vi "Demo.vi"() -> ()   [LabVIEW 2020, in "BlueVariantViewDemo.lvlib"]
uses:
  BlueVariantViewDemo.lvlib
  Classes/Child/Child.lvclass
  C:/DSCE code/Serialization OpenSource/BlueVariantView/Source/Demo/Classes/Parent/Parent.lvclass
  API/Typedefs/Options.ctl
  API/Typedefs/ValueOptions.ctl
  Classes/Parent/Parent.lvclass/Parent.ctl
  Classes/Child/Child.lvclass/Child.ctl
  Classes/Parent/Write connection ID.vi
  Classes/Parent/Write Name.vi
  Classes/Child/Write Color.vi
  Classes/Child/Write Port.vi
  Classes/Child/Write timeout.vi
  BlueVariantView.lvlib
panel:
  out "error out":errorcluster
  in  "Config":T1={"RS232"={"baud rate"=9600, "data bits"=8, "parity"=enum."Even", "stop bits"=10, "flow control"=3, "Numeric"=0.0, "MyRing"=0}, "LEDs"=[FALSE, TRUE, TRUE], "Hazzards"=[{"Alarm"=FALSE, "level"=0.0, "states"=[1, 2, 3]}, {"Alarm"=TRUE, "level"=2.0, "states"=[3, 0, 3, 1]}, {"Alarm"=TRUE, "level"=0.0, "states"=[]}], "Calibration"=[[1.0, 1.2], [2.0, 2.3], [3.0, 3.4]], "MyError"={"status"=FALSE, "code"=123, "source"="This is an error"}, "MyMap"={}, "MySet"={}, "MyVariant"=variant, "MyDVR"=refnum, "MyObject"=refnum, "current time"=timestamp(0 s since 1904-01-01)} {"RS232"."MyRing" items=["a"=3, "b"=4]; "RS232"."flow control" items=["None", "XON/XOFF", "RTS/CTS", "XON/XOFF & RTS/CTS", "DTR/DSR", "XON/XOFF & DTR/DSR"]; "RS232"."stop bits" items=["1.0"=10, "1.5"=15, "2.0"=20]; "RS232"."data bits" min=5 max=8 step=1}
  in  "Tree":string(tree)
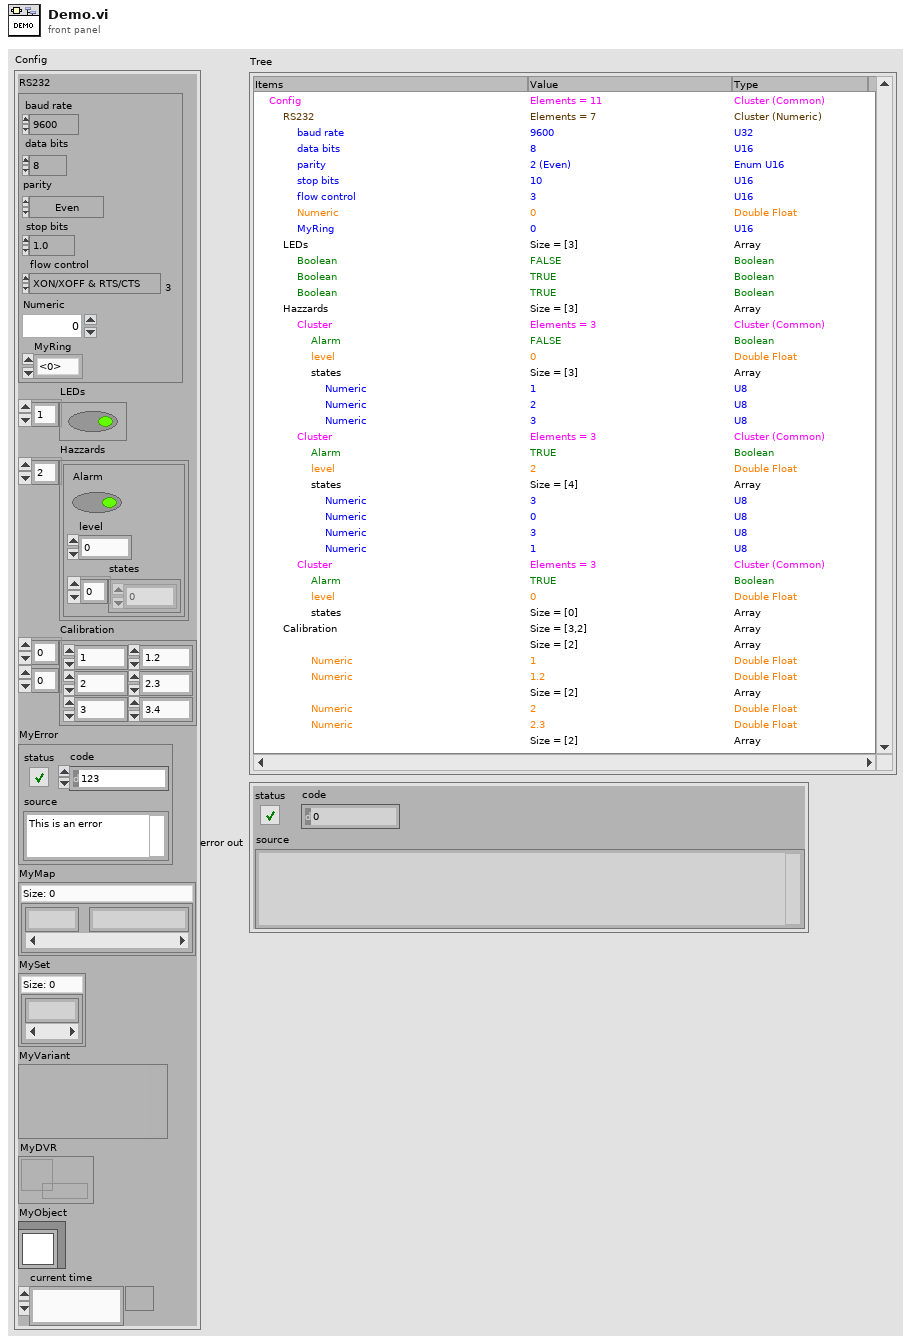
[diagram p1: front panel]
types:
  T1 = cluster{"RS232":cluster{"baud rate":u32, "data bits":u16, "parity":enum16{"None", "Odd", "Even", "Mark", "Space"}, "stop bits":u16, "flow control":u16, "Numeric":dbl, "MyRing":u16}, "LEDs":bool[], "Hazzards":cluster{"Alarm":bool, "level":dbl, "states":u8[]}[], "Calibration":dbl[][], "MyError":errorcluster, "MyMap":map{dbl, string}, "MySet":set{i32}, "MyVariant":variant, "MyDVR":refnum<data-value>, "MyObject":refnum<class "Child.lvclass">, "current time":timestamp}
  T2 = typedef "BlueVariantView.lvlib/ValueOptions.ctl" = enum16{"Verbose", "Data only"}
  T3 = typedef "BlueVariantView.lvlib/Options.ctl" = cluster{"Colorize?":bool, "timestamp format":string, "Value Options":T2}
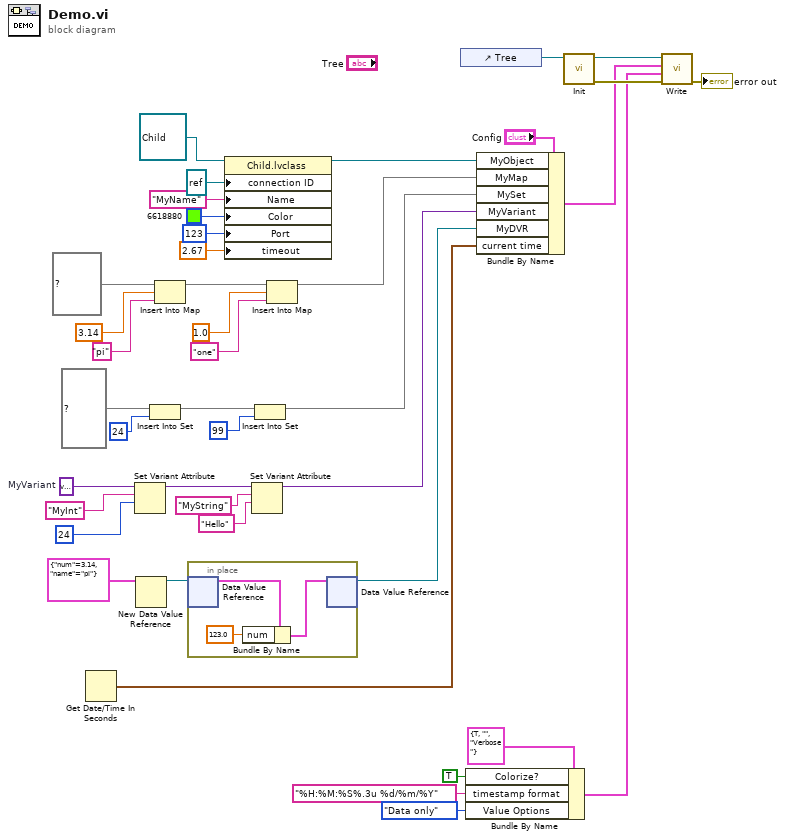
[diagram p0: block diagram]
diagram:
  w27 = variant  # MyVariant
  n1 = Get Date/Time In Seconds() -> (seconds since 1Jan1904=w3:timestamp)
  n2 = Set Variant Attribute(Variant=w27, name="MyInt", value=24 ("element")) -> (Variant out=w24:variant)  [unwired: 1 in, 2 out]
  n3 = New Data Value Reference(data value=cluster{"num":dbl, "name":string} {"num"=3.14, "name"="pi"}) -> (data value reference=w14:refnum<data-value>)  [unwired: 1 in, 1 out]
  n4 = Insert Into Set(10:24 ("element"), 11:set{i32} {} ("set in")) -> (3:w30:set{i32})  [unwired: 1 out]
  n5 = Insert Into Map(map in=map{dbl, string} {} ("MyMap"), key=3.14, value="pi") -> (map out=w36:map{dbl, string})  [unwired: 2 out]
  n6 = in-place {
    n7 = in-place-dvr #1(w14) -> (w44:cluster{"num":dbl, "name":string})  [unwired: 1 out]
    n8 = Bundle By Name(cluster=w44, "num"=123.0) -> (w42:cluster{"num":dbl, "name":string})
    n9 = in-place-dvr #1(w42) -> (w13:refnum<data-value>)  [unwired: 1 out]
  }
  n10 = property class="Child.lvclass"(reference=refnum<class "Child.lvclass"> refnum ("BlueVariantViewDemo.lvlib:Child.lvclass"), "connection ID"=refnum<k5> refnum, "Name"="MyName", "Color"=u32 6618880, "Port"=123, "timeout"=2.67) -> (reference out=w40:refnum<class "Child.lvclass">)  [unwired: 1 in, 1 out]
  n11 = Set Variant Attribute(Variant=w24, name="MyString", value="Hello" ("name")) -> (Variant out=w21:variant)  [unwired: 1 in, 2 out]
  n12 = Insert Into Set(10:99 ("element"), 11:w30) -> (3:w28:set{i32})  [unwired: 1 out]
  n13 = Insert Into Map(map in=w36, key=1.0, value="one") -> (map out=w33:map{dbl, string})  [unwired: 2 out]
  n14 = control-ref of="Tree"() -> (w17:refnum<vi>)
  n15 = Bundle By Name(cluster=T3 {"Colorize?"=TRUE, "timestamp format"="", "Value Options"=enum."Verbose"} ("Options"), "Colorize?"=TRUE, "timestamp format"="%H:%M:%S%.3u %d/%m/%Y", "Value Options"=ValueOptions."Data only") -> (w10:T3)
  n16 = Bundle By Name(cluster="Config", "MyObject"=w40, "MyMap"=w33, "MySet"=w28, "MyVariant"=w21, "MyDVR"=w13, "current time"=w3) -> (w16:T1)
  n17 = call "Init.vi"("Tree in"=w17) -> ("error out"=w18:errorcluster, "Tree out"=w19:refnum<vi>)  [unwired: 9 in]
  n18 = call "Write.vi"("error in (no error)"=w18, "Options"=w10, "Anything"=w16, "Tree in"=w19) -> ("error out"=→"error out":errorcluster)  [unwired: 5 in, 2 out]
